vi "GetClientInfo.vi"() -> (0 "IsClient":bool, 1 "Produce Read Errors":bool, 2 "Start Time":string, 3 "Name":string, 4 "ValidateTable":bool, 5 "Variable Count":i32, 6 "ConnectionNames":string[](array[string]), 7 "ConnectionCount":i32, 8 "InitComplete":bool[](array[boolean]))   [LabVIEW 2019]
uses:
  <vilib>/Rock Robotics/Network Tables/NT Globals.vi
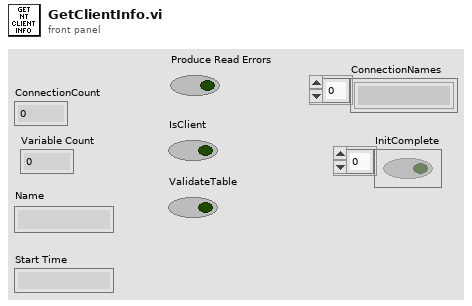
[diagram p1: front panel]
types:
  T1 = enum16{"Add Cnx", "Remove Cnx", "Retrieve List", "Cnx Inited"}
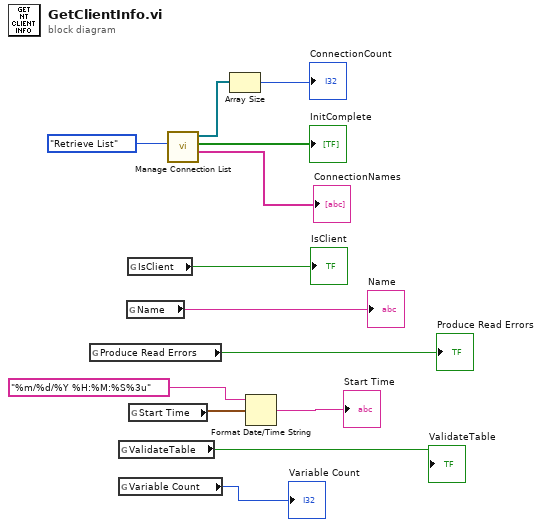
[diagram p0: block diagram]
diagram:
  n1 = global read "NT Globals.vi" "Produce Read Errors"() -> (→"Produce Read Errors":bool)
  n2 = global read "NT Globals.vi" "ValidateTable"() -> (→"ValidateTable":bool)
  n3 = global read "NT Globals.vi" "Variable Count"() -> (→"Variable Count":i32)
  n4 = global read "NT Globals.vi" "Name"() -> (→"Name":string)
  n5 = global read "NT Globals.vi" "IsClient"() -> (→"IsClient":bool)
  n6 = global read "NT Globals.vi" "Start Time"() -> (w7:timestamp)
  n7 = call <vilib>:"Manage Connection List.vi"("Operation"=T1."Retrieve List") -> ("Names"=→"ConnectionNames":string[], "Inited"=→"InitComplete":bool[], "Connections List"=w12:refnum<k5>[])  [unwired: 8 in]
  n8 = Array Size(array=w12) -> (size(s)=→"ConnectionCount":i32)
  n9 = Format Date/Time String(time format string (%c)="%m/%d/%Y %H:%M:%S%3u", seconds (now)=w7) -> (date/time string=→"Start Time":string)  [unwired: 1 in]
